vi "Ramsete Controller.vi"(8 "Turing Parameters":cluster{"b":dbl, "zeta":dbl}={"b"=2.0, "zeta"=0.7}, 9 "Velocity Ref":T1 {"Angular Velocity Ref" format="%#_13g"; "Linear Velocity Ref" format="%#_13g"}, 10 "Pose Ref":T2, 11 "Current Pose":T2) -> (2 "Angular Velocity":dbl, 3 "Linear Velocity":dbl)   [LabVIEW 2019]
uses:
  Geometry/Typedef/Pose2d.ctl
  Geometry/Typedef/Translation2d.ctl
  Geometry/Typedef/Rotation2d.ctl
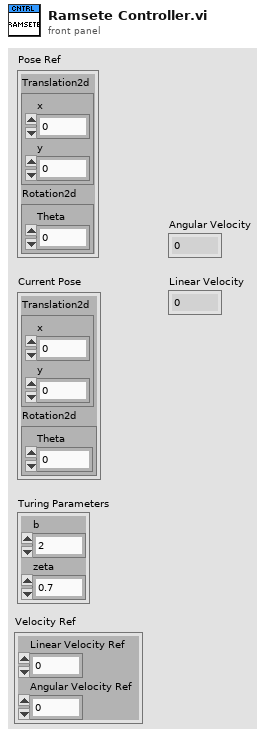
[diagram p1: front panel]
types:
  T1 = cluster{"Linear Velocity Ref":dbl, "Angular Velocity Ref":dbl}
  T2 = typedef "Pose2d.ctl" = cluster{"Translation2d":T3, "Rotation2d":T4}
  T3 = typedef "Translation2d.ctl" = cluster{"x":dbl, "y":dbl}
  T4 = typedef "Rotation2d.ctl" = cluster{"Theta":dbl}
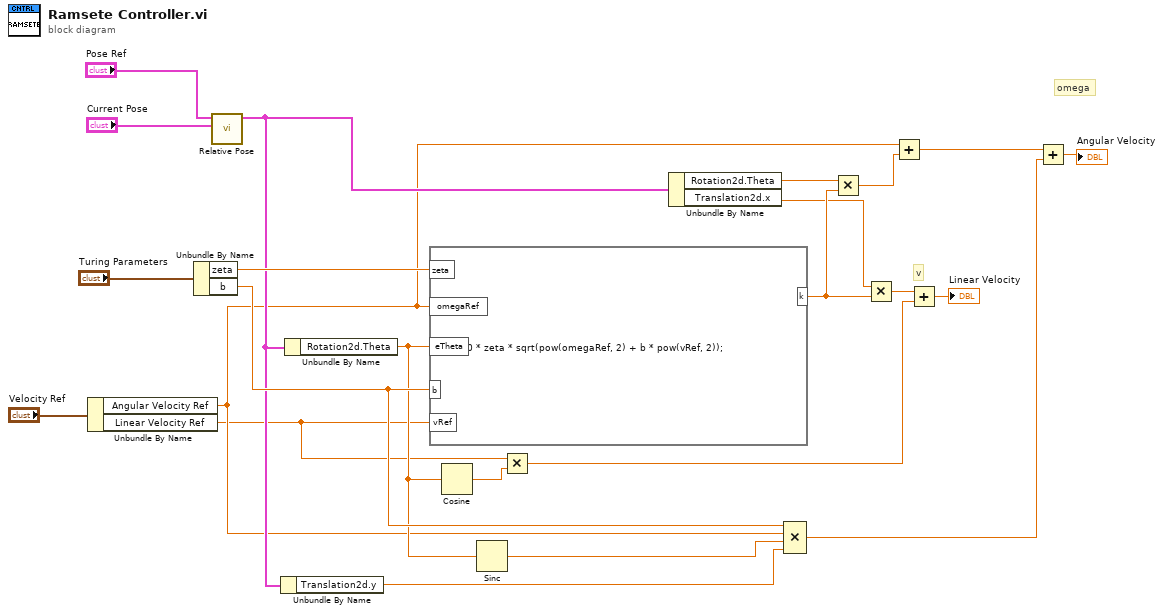
[diagram p0: block diagram]
diagram:
  # "omega"
  # "v"
  n1 = Unbundle By Name("Velocity Ref") -> ("Angular Velocity Ref"=w2:dbl, "Linear Velocity Ref"=w1:dbl)
  n2 = Unbundle By Name("Turing Parameters") -> ("zeta"=w23:dbl, "b"=w22:dbl)
  n3 = call "Relative Pose.vi"("Final"="Current Pose", "Initial"="Pose Ref") -> ("Relative Pose"=w13:T2)  [unwired: 9 in]
  n4 = Unbundle By Name(w13) -> ("Translation2d.y"=w14:dbl)
  n5 = Unbundle By Name(w13) -> ("Rotation2d.Theta"=w15:dbl)
  n6 = formula code="k = 2.0 * zeta * sqrt(pow(omegaRef, 2) + b * pow(vRef, 2));"("zeta"=w23, "omegaRef"=w2, "eTheta"=w15, "b"=w22, "vRef"=w1) -> ("k"=w10:dbl)
  n7 = Cosine(x=w15) -> (cos(x)=w6:dbl)
  n8 = Sinc(1:w15) -> (0:w16:dbl)
  n9 = Multiply(x=w1, y=w6) -> (x*y=w7:dbl)
  n10 = Unbundle By Name(w13) -> ("Rotation2d.Theta"=w11:dbl, "Translation2d.x"=w8:dbl)
  n11 = Compound Arithmetic op=MULTIPLY(w22, w2, w16, w14) -> (w18:dbl)
  n12 = Multiply(x=w11, y=w10) -> (x*y=w12:dbl)
  n13 = Multiply(x=w8, y=w10) -> (x*y=w9:dbl)
  n14 = Add(x=w2, y=w12) -> (x+y=w17:dbl)
  n15 = Add(x=w9, y=w7) -> (x+y=→"Linear Velocity":dbl)
  n16 = Add(x=w17, y=w18) -> (x+y=→"Angular Velocity":dbl)
